vi "ZMC Up3File.vi"(8 "error in (no error)":errorcluster caption="错误输入（无错误）", 9 "pfilenameinControl":string, 10 "pfilename":string, 11 "handle":u32) -> (0 "error out":errorcluster caption="错误输出", 2 "function return":i32, 3 "handle out":u32)   [LabVIEW 2015, in "zauxdll.lvlib"]
doc: "int32 __stdcall ZMC_Up3File(ZMC_HANDLE handle, const char* pfilename, const char* pfilenameinControl);"
uses:
  zauxdll.lvlib
  zmotion.dll
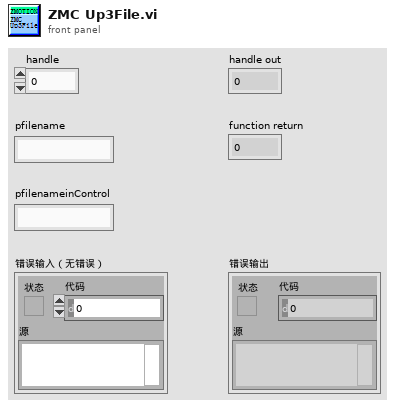
[diagram p1: front panel]
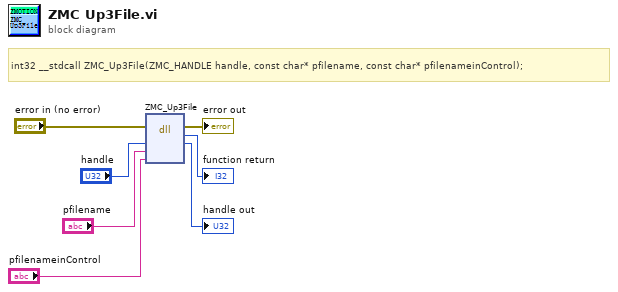
[diagram p0: block diagram]
diagram:
  # "int32 __stdcall ZMC_Up3File(ZMC_HANDLE handle, const char* pfilename, const char* pfilenameinControl);"
  n1 = dll-call lib="C:/Users/VIC/Desktop/GOGORO_SA/system/LLB/zmotion/zaux/zmotion.*" fn="ZMC_Up3File"(error in="error in (no error)", "handle"="handle", "pfilename"="pfilename", "pfilenameinControl"="pfilenameinControl") -> (error out=→"error out":errorcluster, →"function return":i32, "handle"=→"handle out":u32)  [unwired: 4 in, 1 out]
